vi "CommonVIs_ClassWireSelection.vi"(3 "Offset(-300,0)":T1={"Left"=-231, "Top"=18}, 4 "SaveChangesInClassRightAway(True)":bool=TRUE, 5 "WireStyleSelected":refnum<user-event>, 7 "SelectedWireStyle":refnum<vi>, 8 "error in (no error)":errorcluster, 9 "Messages(Stop or Empty string will stop this VI)":refnum<user-event>, 10 "WireSelectionList":refnum<vi>, 11 "LVClassToActOn":refnum<vi>) -> ()   [LabVIEW 2020]
uses:
  <vilib>/Utility/miscctls.llb/LVPositionTypeDef.ctl
  <resource>/Framework/Providers/Open_GDS/SubVIs/GOOP_WireConfigurationType.ctl
  <resource>/Framework/Providers/Open_GDS/SubVIs/GOOP_WirePattern.ctl
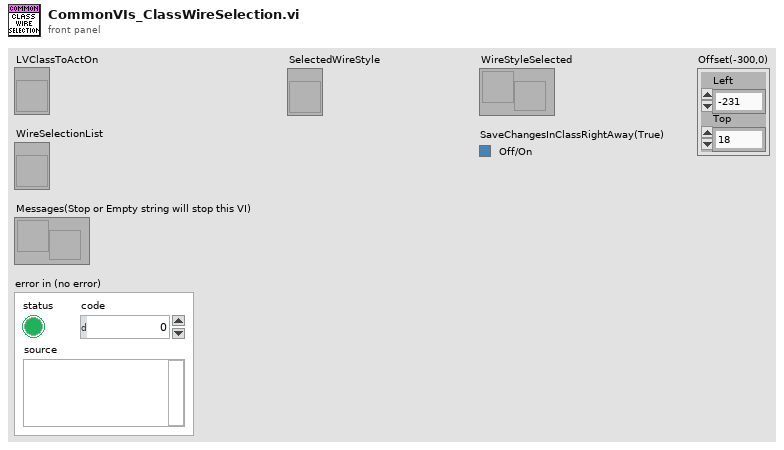
[diagram p1: front panel]
types:
  T1 = typedef "LVPositionTypeDef.ctl" = cluster{"Left":i32, "Top":i32}
  T2 = typedef "GOOP_WireConfigurationType.ctl" = cluster{"Edge thickness":i32, "Edge color":u32, "Center thickness":i32, "Center pattern":T3, "CenterColor1":u32, "CenterColor2":u32, "Tunnels and terminals colors":u32}
  T3 = typedef "GOOP_WirePattern.ctl" = enum16{"Solid", "Large dash", "Small dash"}
  T4 = cluster{"SelectedWireStyle":string, "IconSelection":picture, "CurrentWire":picture, "Icons":string[][], "MarkedIconSelection":picture, "Timeout":i32, "SelectedWireStyle":T2}
  T5 = cluster{"Width":i16, "Style":enum32{"Solid", "Dash", "Dot", "DashDot", "DashDotDot"}}
  T6 = cluster{"left":i16, "top":i16, "right":i16, "bottom":i16}
  T7 = cluster{"IconDimensions":i16, "IconDimensions":i16}
  T8 = cluster{"Foreground Color":u32, "Background Color":u32, "Fill Pattern":cluster{"Row 0":u8, "Row 1":u8, "Row 2":u8, "Row 3":u8, "Row 4":u8, "Row 5":u8, "Row 6":u8, "Row 7":u8}, "Width":i16, "Mode":enum16{"Copy", "Or", "Exclusive Or", "Bit Clear", "Not Copy", "Not Or", "Nor Exclusive Or", "Not Bit Clear"}, "Style":enum32{"Solid", "Dash", "Dot", "Dash Dot", "Dash Dot Dot"}, "Fill Rule":enum32{"Even Odd", "Winding"}, "End Caps":enum32{"Default", "Flat"}}[]
  T9 = typedef "lveventtype.ctl" = enum32{"Null", "Timeout", "Annotation Menu Selection", "Annotation Menu Selection?", "App Instance Close", "App Instance Close?", "Autoscale Range Change", "Bookmark Info Change", "Cell Edit", "Cell Edit?", "Cursor Grab", "Cursor Grab?", "Cursor Menu Selection", "Cursor Menu Selection?", "Cursor Move", "Cursor Release", "Data Change", "Direction Change", "Display State Change", "Drag Ended", "Drag Enter", "Drag Leave", "Drag Over", "Drag Source Update", "Drag Starting", "Drag Starting?", "Drop", "Exec State Change", "Key Down", "Key Down?", "Key Repeat", "Key Repeat?", "Key Up", "Listbox Double Click", "Menu Activation?", "Menu Selection (App)", "Menu Selection? (App)", "Menu Selection (User)", "Mouse Down", "Mouse Down?", "Mouse Enter", "Mouse Leave", "Mouse Move", "Mouse Up", "Mouse Wheel", "NI Security User Change (App)", "Pane Size", "Panel Close", "Panel Close?", "Panel Resize", "Plot Attribute Change", "Scale Range Change", "Shortcut Menu Activation?", "Shortcut Menu Selection (App)", "Shortcut Menu Selection? (App)", "Shortcut Menu Selection (User)", "Tree Double Click", "Tree Drag", "Tree Drag?", "Tree Drop", "Tree Drop?", "Tree Item Close", "Tree Item Close?", "Tree Item Open", "Tree Item Open?", "User Event", "Value Change"}
  T10 = cluster{"IconDimensions":i16, "IconDimensions":i16, "IconDimensions":i16, "IconDimensions":i16}
  T11 = cluster{"IconDimensions":dbl, "IconDimensions":dbl}
  T12 = cluster{"IconDimensions":i32, "IconDimensions":i32}
  T13 = cluster{"IconDimensions":i32, "IconDimensions":i32, "IconDimensions":i32, "IconDimensions":i32}
  T14 = typedef "Scripting_ConnectorPanePatternType.ctl" = u16
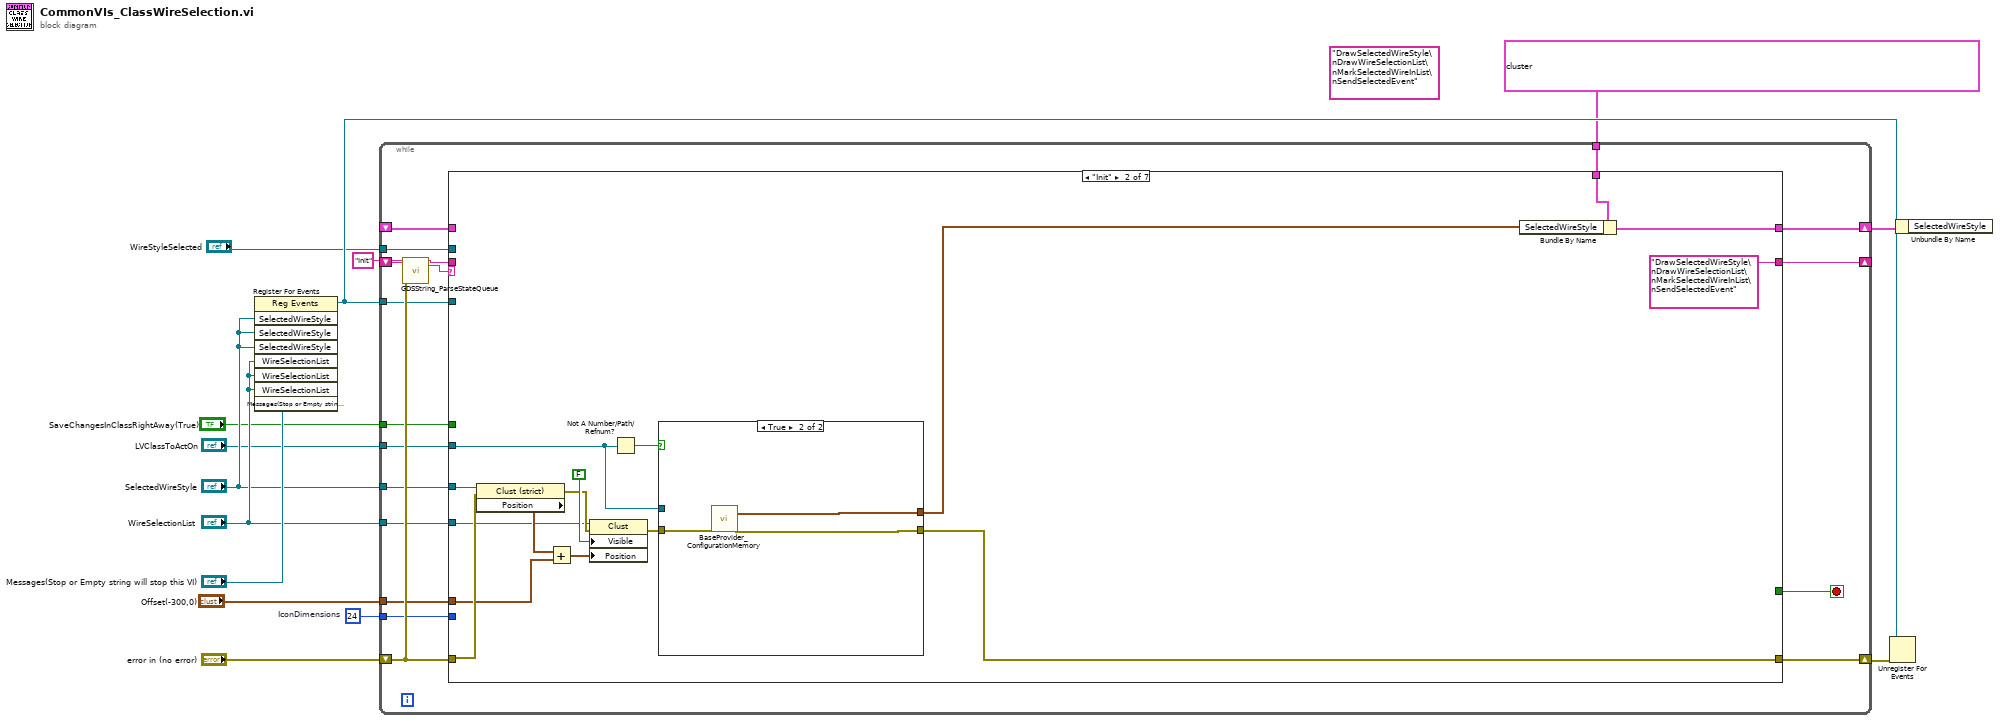
[diagram p0: block diagram]
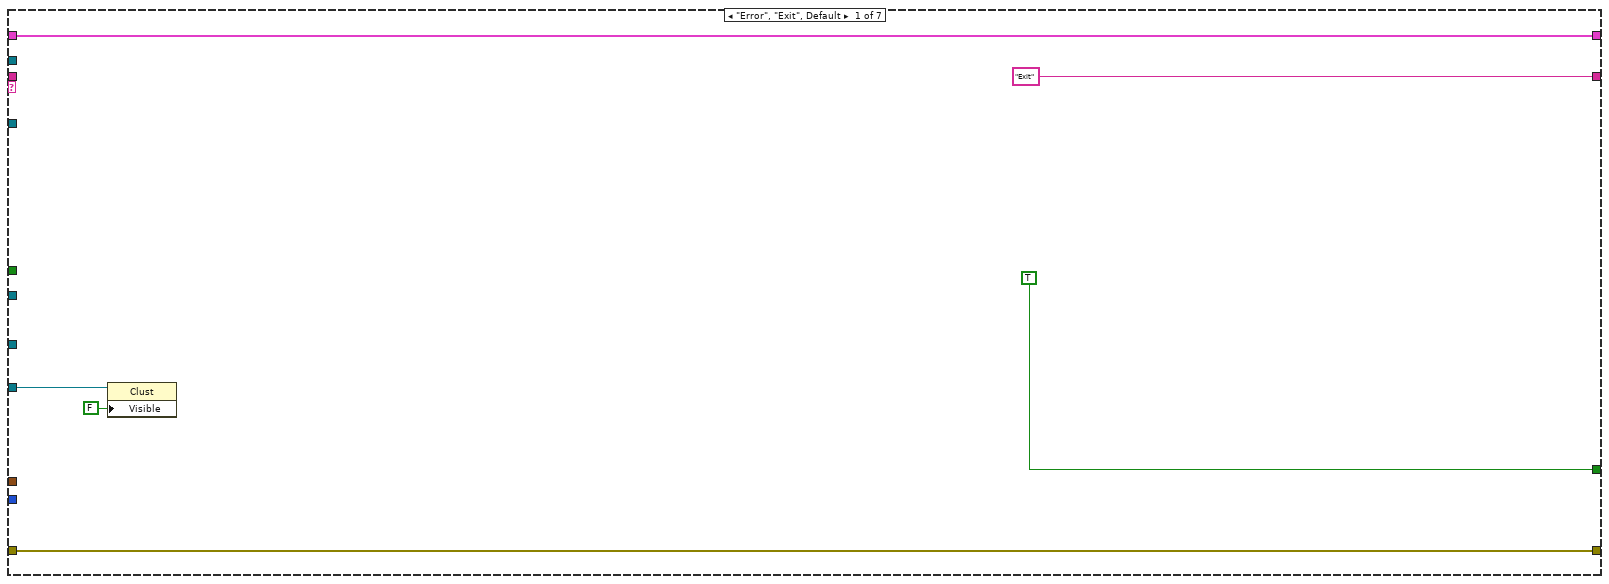
[diagram p2: hidden frame]
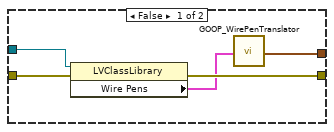
[diagram p3: hidden frame]
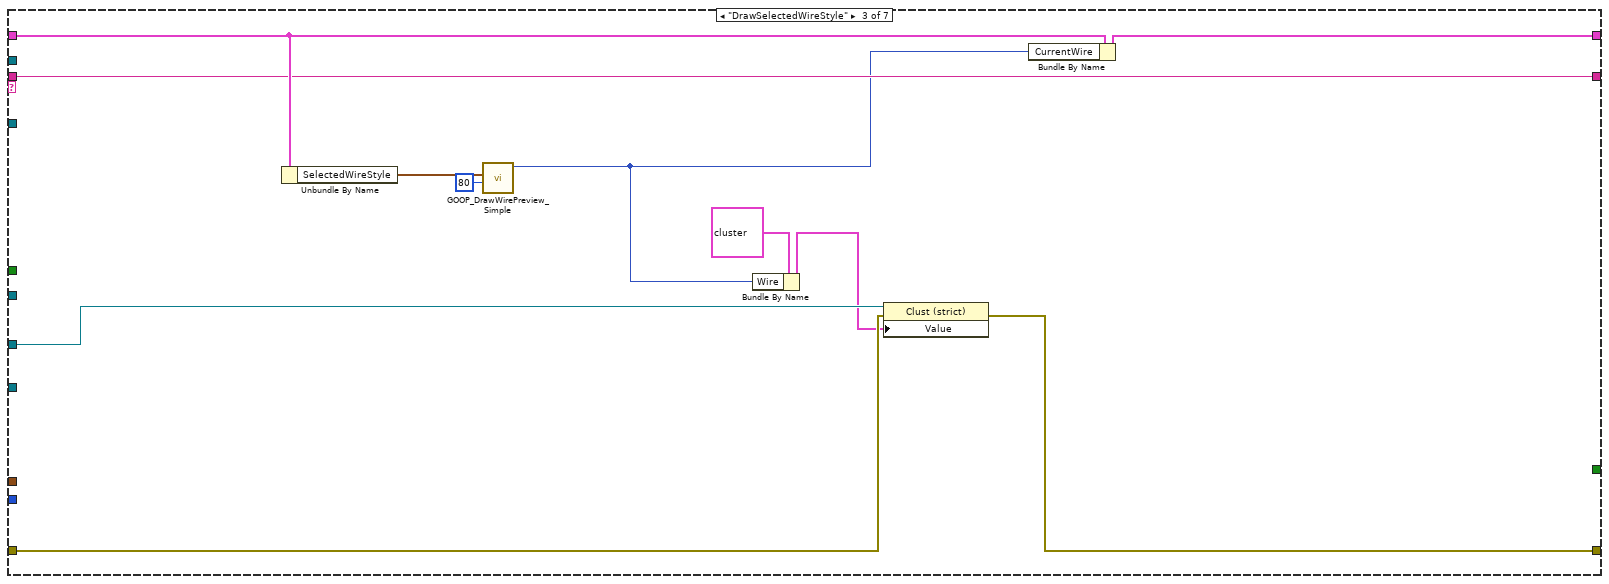
[diagram p4: hidden frame]
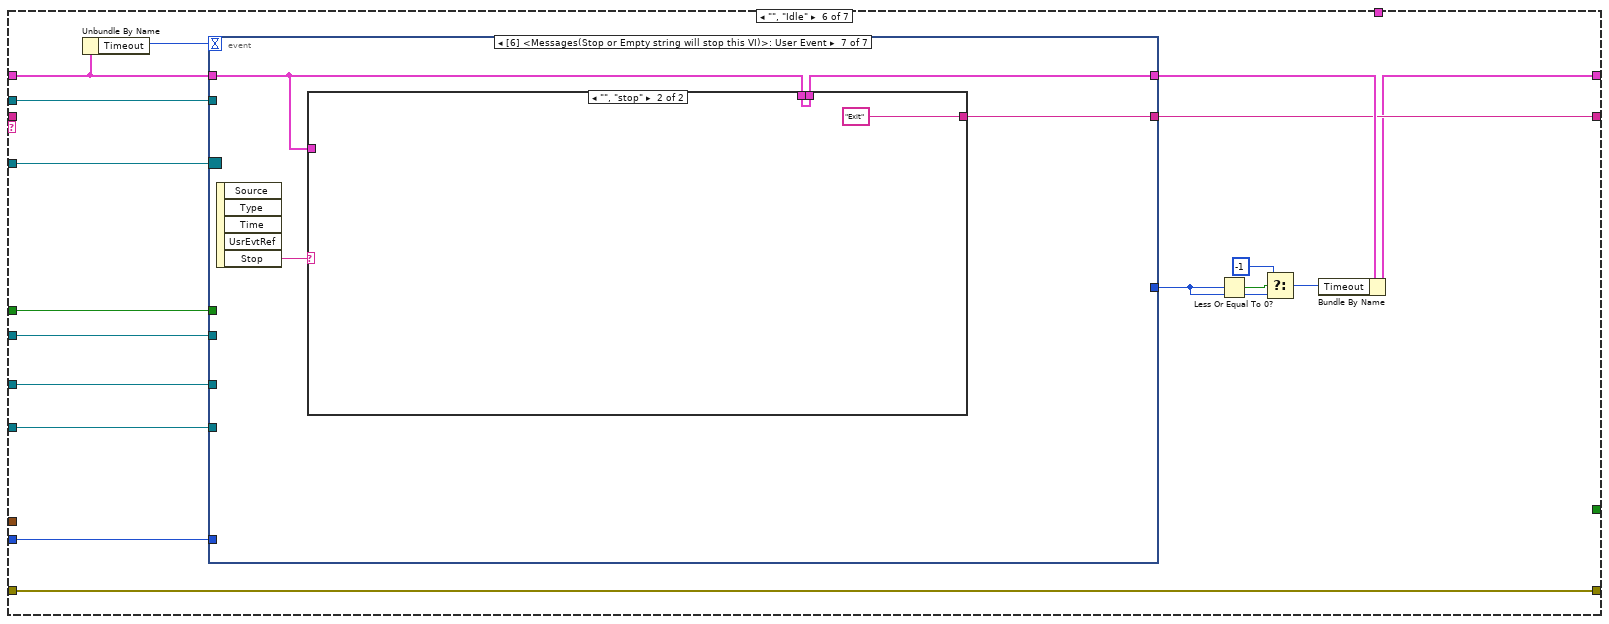
[diagram p7: hidden frame]
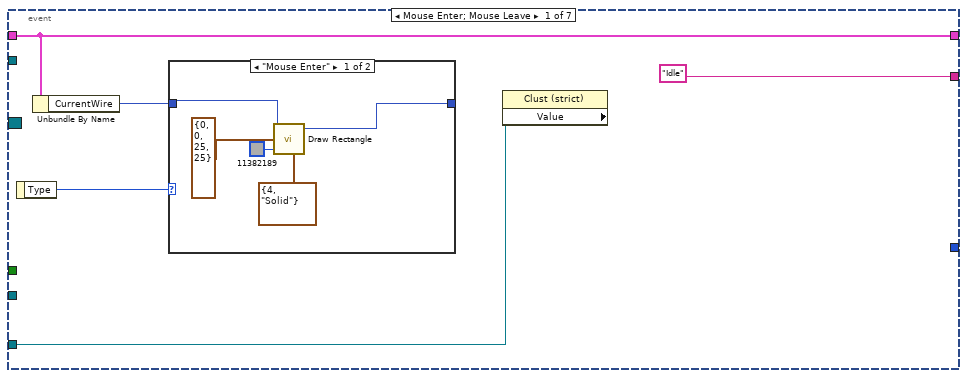
[diagram p8: hidden frame]
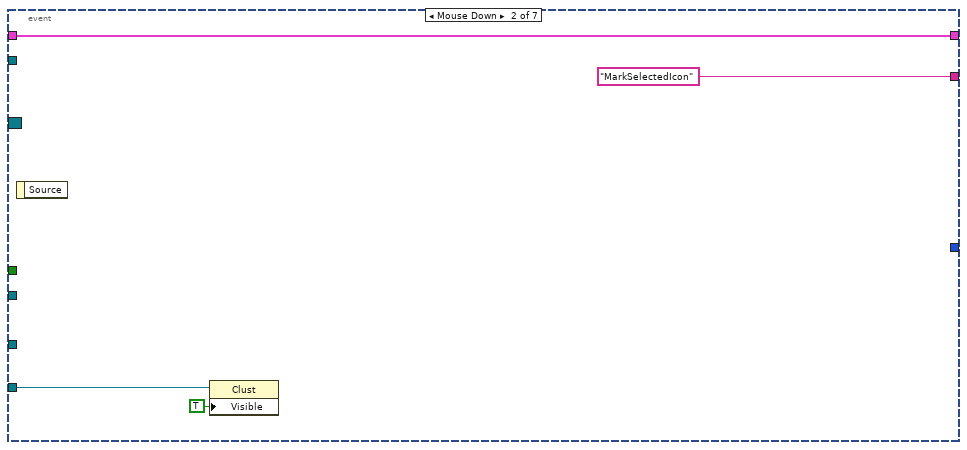
[diagram p10: hidden frame]
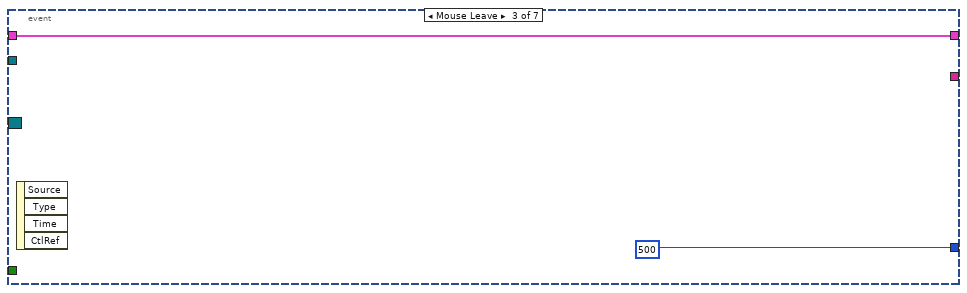
[diagram p11: hidden frame]
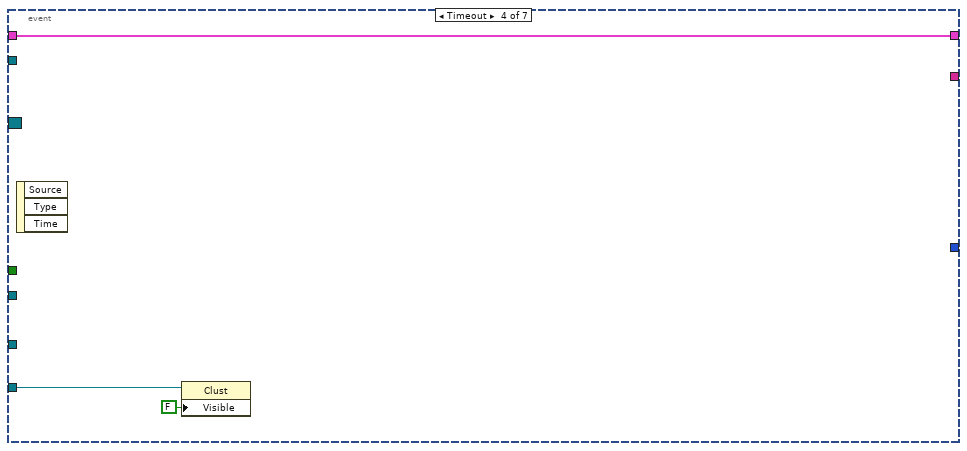
[diagram p12: hidden frame]
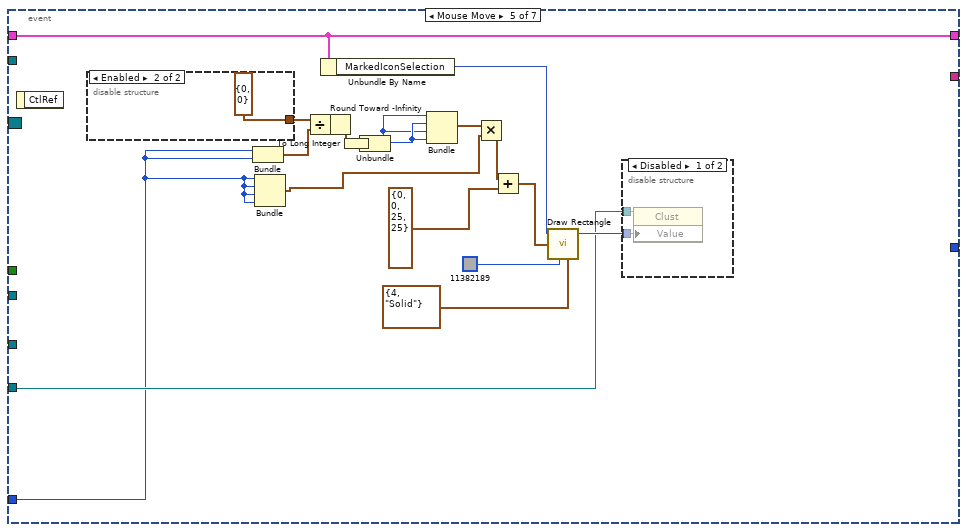
[diagram p13: hidden frame]
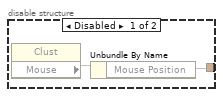
[diagram p15: hidden frame]
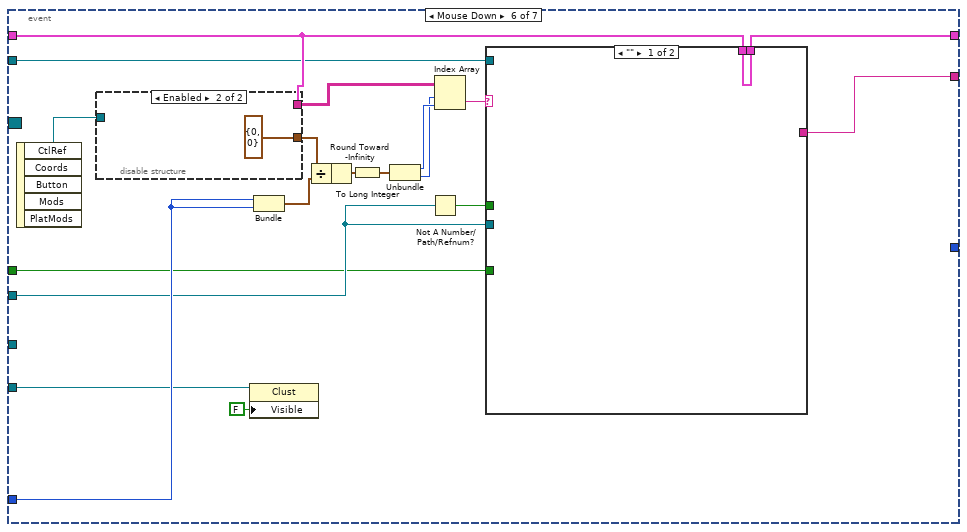
[diagram p16: hidden frame]
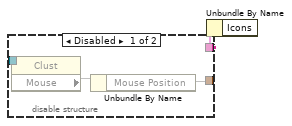
[diagram p17: hidden frame]
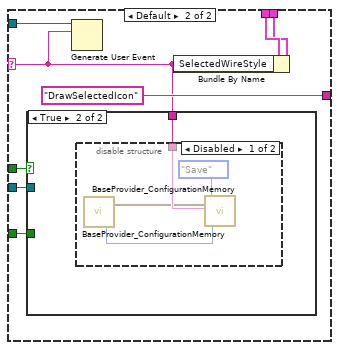
[diagram p18: hidden frame]
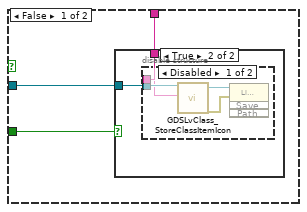
[diagram p19: hidden frame]
diagram:
  (unwired) "DrawSelectedWireStyle\nDrawWireSelectionList\nMarkSelectedWireInList\nSendSelectedEvent"
  w7 = i16 24  # IconDimensions
  n1 = register-events("SelectedWireStyle", "SelectedWireStyle", "SelectedWireStyle", "WireSelectionList", "WireSelectionList", "WireSelectionList", "Messages(Stop or Empty string will stop this VI)") -> (reference out=w11:refnum<event-registration>)  [unwired: 2 in, 1 out]
  n2 = while {
    shift-right: [w28] -> w10
    shift-left: "error in (no error)" -> [w31]
    shift-right: [w27] -> _
    shift-left: "Init" -> [w32]
    tunnel: "WireSelectionList" -> [w30]
    tunnel: "SelectedWireStyle" -> [w29]
    tunnel: w7 -> [w23]
    tunnel: T4 {"SelectedWireStyle"="", "IconSelection"=bytes[0], "CurrentWire"=bytes[0], "Icons"=[], "MarkedIconSelection"=bytes[0], "Timeout"=-1, "SelectedWireStyle"={"Edge thickness"=1, "Edge color"=5667411, "Center thickness"=1, "Center pattern"=enum."Solid", "CenterColor1"=9740924, "CenterColor2"=8694662, "Tunnels and terminals colors"=131187}} -> [w22]
    shift-right: [w21] -> w13
    shift-left: _ -> [w20]
    tunnel: w11 -> [w19]
    tunnel: "LVClassToActOn" -> [w18]
    tunnel: "WireStyleSelected" -> [w17]
    tunnel: "SaveChangesInClassRightAway(True)" -> [w16]
    tunnel: "Offset(-300,0)" -> [w15]
    stop <- w26 stop-if-true
    n3 = call <resource>:"GDSString_ParseStateQueue.vi"("State Queue"=w32, "Error In (no error)"=w31) -> ("Remaining States"=w25:string, "Current State"=w24:string)  [unwired: 9 in, 3 out]
    n4 = case shown="\"Init\"" w24 {
      tunnel: w31 -> [w38 w52 w67 w76 w78 w96 w216]
      tunnel: w30 -> [w34 w46 _ _ _ w92 _]
      tunnel: w29 -> [_ w47 w69 _ _ w83 _]
      tunnel: [w38 w45 w72 w76 w78 w96 w216] -> w28
      tunnel: ["Exit" "DrawSelectedWireStyle\nDrawWireSelectionList\nMarkSelectedWireInList\nSendSelectedEvent" w70 w75 w79 w93 w215] -> w27
      tunnel: [TRUE _ _ _ _ _ _] -> w26
      tunnel: w25 -> [_ _ w70 w75 w79 _ w215]
      tunnel: w23 -> [_ _ _ _ _ w91 _]
      tunnel: w22 -> [_ w49 _ _ _ _ _]
      tunnel: [w35 w48 w71 w74 w77 w90 w213] -> w21
      tunnel: w20 -> [w35 _ w73 w74 w77 w85 w213]
      tunnel: w19 -> [_ _ _ _ _ w95 _]
      tunnel: w18 -> [_ w42 _ _ _ w82 _]
      tunnel: w17 -> [_ _ _ _ _ w81 w214]
      tunnel: w16 -> [_ _ _ _ _ w80 _]
      tunnel: w15 -> [_ w39 _ _ _ _ _]
      frame "Error", "Exit", Default {
        n5 = property class="Clust"(reference=w34, "Visible"=FALSE) -> ()  [unwired: 1 in, 2 out]
      }
      frame "Init" {
        n6 = property class="Clust (strict)"(reference=w47, error in=w52) -> (error out=w51:errorcluster, "Position"=w54:T1)  [unwired: 1 out]
        n7 = Add(x=w54, y=w39) -> (x+y=w40:T1)
        n8 = property class="Clust"(reference=w46, error in=w51, "Visible"=FALSE, "Position"=w40) -> (error out=w50:errorcluster)  [unwired: 1 out]
        n9 = Not A Number/Path/Refnum?(number/path/refnum=w42) -> (NaN/Path/Refnum?=w43:bool)
        n10 = case shown="True" w43 {
          tunnel: w50 -> [w58 w62]
          tunnel: [w57 w61] -> w45
          tunnel: [w56 w60] -> w44
          tunnel: w42 -> [w59 _]
          frame False {
            n11 = property class="LVClassLibrary"(reference=w59, error in=w58) -> (error out=w57:errorcluster, "Wire Pens"=w55:T8)  [unwired: 1 out]
            n12 = call <resource>:"GOOP_WirePenTranslator.vi"("WirePensIn"=w55) -> ("WireConfigurationOut"=w56:T2)  [unwired: 17 in, 1 out]
          }
          frame True {
            n13 = call <resource>:"BaseProvider_ConfigurationMemory.vi"("error in (no error)"=w62) -> ("WireConfigurationOut"=w60:T2, "error out"=w61:errorcluster)  [unwired: 12 in, 5 out]
          }
        }
        n14 = Bundle By Name(cluster=w49, "SelectedWireStyle"=w44) -> (w48:T4)
      }
      frame "DrawSelectedWireStyle" {
        n15 = Unbundle By Name(w73) -> ("SelectedWireStyle"=w68:T2)
        n16 = call <resource>:"GOOP_DrawWirePreview_Simple.vi"("WireLength(100px)"=i16 80, "WireConfiguration"=w68) -> ("WirePictureOut"=w64:picture)  [unwired: 5 in, 4 out]
        n17 = Bundle By Name(cluster=cluster{"Name":string, "Wire":picture} {"Name"="Default", "Wire"=bytes[0]} ("Value"), "Wire"=w64) -> (w65:cluster{"Name":string, "Wire":picture})
        n18 = property class="Clust (strict)"(reference=w69, error in=w67, "Value"=w65) -> (error out=w72:errorcluster)  [unwired: 1 out]
        n19 = Bundle By Name(cluster=w73, "CurrentWire"=w64) -> (w71:T4)
      }
      frame "DrawWireSelectionList" {
      }
      frame "MarkSelectedWireInList" {
      }
      frame "", "Idle" {
        n20 = Unbundle By Name(w85) -> ("Timeout"=w84:i32)
        n21 = event shown="[6] <Messages(Stop or Empty string will stop this VI)>: User Event" {
          selector: w95 -> [_ _ _ _ _ _ _]
          dyn-events: _ -> [_ _ _ _ _ _ _]
          timeout: w84 -> [_ _ _ _ _ _ _]
          tunnel: w85 -> [w100 w109 w113 w116 w122 w153 w190]
          tunnel: [w100 w109 w113 w116 w122 w151 w191] -> w94
          tunnel: ["Idle" "MarkSelectedIcon" _ _ _ w149 w192] -> w93
          tunnel: w92 -> [_ w111 _ w114 w119 w147 _]
          tunnel: w91 -> [_ _ _ _ w118 w154 _]
          tunnel: [_ _ 500 ("500") _ _ _ _] -> w87
          tunnel: w83 -> [w97 _ _ _ _ _ _]
          tunnel: w82 -> [_ _ _ _ _ w143 _]
          tunnel: w81 -> [_ _ _ _ _ w142 _]
          tunnel: w80 -> [_ _ _ _ _ w141 _]
          event Mouse Enter; Mouse Leave {
            n22 = event-data() -> ("Type"=w101:T9)  [unwired: 1 in]
            n23 = Unbundle By Name(w100) -> ("CurrentWire"=w99:picture)
            n24 = case shown="\"Mouse Enter\"" w101 {
              tunnel: [w104 w107] -> _
              tunnel: w99 -> [w103 w107]
              frame "Mouse Enter" {
                n25 = call <vilib>:"Draw Rectangle.vi"("picture"=w103, "rect"=T6 {"left"=0, "top"=0, "right"=25, "bottom"=25}, "color(black)"=u32 11382189, "pen"=T5 {"Width"=4, "Style"=enum."Solid"}) -> ("new picture"=w104:picture)  [unwired: 5 in]
              }
              frame "Mouse Leave", Default {
              }
            }
            n26 = property class="Clust (strict)" props=["Value"](reference=w97) -> ()  [unwired: 1 in, 3 out]
          }
          event Mouse Down {
            n27 = event-data() -> ()  [unwired: 1 in, 1 out]
            n28 = property class="Clust"(reference=w111, "Visible"=TRUE) -> ()  [unwired: 1 in, 2 out]
          }
          event Mouse Leave {
            n29 = event-data() -> ()  [unwired: 1 in, 4 out]
          }
          event Timeout {
            n30 = event-data() -> ()  [unwired: 1 in, 3 out]
            n31 = property class="Clust"(reference=w114, "Visible"=FALSE) -> ()  [unwired: 1 in, 2 out]
          }
          event Mouse Move {
            n32 = event-data() -> ()  [unwired: 1 in, 1 out]
            n33 = disable-structure shown="Enabled" {
              disable-tunnel: [w139 T7 {"IconDimensions"=0, "IconDimensions"=0} ("x")] -> w124
              frame Disabled {
                n34 = property on="Property Node" class="Clust"() -> ("Mouse"=w138)  [unwired: 2 in, 2 out]
                n35 = Unbundle By Name(w138) -> ("Mouse Position"=w139)
              }
              frame Enabled {
              }
            }
            n36 = Bundle("IconDimensions"=w118, "IconDimensions"=w118) -> (w123:T7)  [unwired: 1 in]
            n37 = Bundle("IconDimensions"=w118, "IconDimensions"=w118, "IconDimensions"=w118, "IconDimensions"=w118) -> (w117:T10)  [unwired: 1 in]
            n38 = Divide(x=w124, y=w123) -> (x/y=w125:T11)
            n39 = Unbundle By Name(w122) -> ("MarkedIconSelection"=w121:picture)
            n40 = Round Toward -Infinity(1:w125) -> (0:w126:T11)
            n41 = To Long Integer(number=w126) -> (32bit integer=w131:T12)
            n42 = Unbundle(w131) -> ("IconDimensions"=w129:i32, "IconDimensions"=w130:i32)
            n43 = Bundle("IconDimensions"=w129, "IconDimensions"=w130, "IconDimensions"=w129, "IconDimensions"=w130) -> (w132:T13)  [unwired: 1 in]
            n44 = Multiply(x=w132, y=w117) -> (x*y=w134:T13)
            n45 = Add(x=w134, y=T6 {"left"=0, "top"=0, "right"=25, "bottom"=25} ("rect")) -> (x+y=w135:cluster{i32, i32, i32, i32})
            n46 = call <vilib>:"Draw Rectangle.vi"("picture"=w121, "rect"=w135, "color(black)"=u32 11382189, "pen"=T5 {"Width"=4, "Style"=enum."Solid"}) -> ("new picture"=w120:picture)  [unwired: 5 in]
            n47 = disable-structure shown="Disabled" {
              disable-tunnel: w120 -> [w137 _]
              disable-tunnel: w119 -> [w136 _]
              frame Disabled {
                n48 = property class="Clust"(reference=w136, "Value"=w137) -> ()  [unwired: 1 in, 2 out]
              }
              frame Enabled {
              }
            }
          }
          event Mouse Down {
            n49 = event-data() -> ("CtlRef"=w155:refnum<vi>)  [unwired: 1 in, 4 out]
            n50 = disable-structure shown="Enabled" {
              disable-tunnel: [w165 T7 {"IconDimensions"=0, "IconDimensions"=0} ("x")] -> w157
              disable-tunnel: w155 -> [w163 _]
              disable-tunnel: w153 -> [w162 _]
              disable-tunnel: [w161 _] -> w152
              frame Disabled {
                n51 = property on="Property Node" class="Clust"(reference=w163) -> ("Mouse"=w164)  [unwired: 1 in, 2 out]
                n52 = Unbundle By Name(w164) -> ("Mouse Position"=w165)
                n53 = Unbundle By Name(w162) -> ("Icons"=w161:string[][])
              }
              frame Enabled {
              }
            }
            n54 = property class="Clust"(reference=w147, "Visible"=FALSE) -> ()  [unwired: 1 in, 2 out]
            n55 = Bundle("IconDimensions"=w154, "IconDimensions"=w154) -> (w156:T7)  [unwired: 1 in]
            n56 = Divide(x=w157, y=w156) -> (x/y=w158:T11)
            n57 = Round Toward -Infinity(1:w158) -> (0:w159:T11)
            n58 = To Long Integer(number=w159) -> (32bit integer=w160:T12)
            n59 = Unbundle(w160) -> ("IconDimensions"=w146:i32, "IconDimensions"=w145:i32)
            n60 = Not A Number/Path/Refnum?(number/path/refnum=w143) -> (NaN/Path/Refnum?=w144:bool)
            n61 = Index Array(array=w152, index (row)=w145, index (col)=w146) -> (element=w150:string)
            n62 = case shown="\"\"" w150 {
              selector: w150 -> [_ w170]
              tunnel: w153 -> [w167 w175]
              tunnel: [w167 w174] -> w151
              tunnel: [_ "DrawSelectedIcon"] -> w149
              tunnel: w144 -> [_ w172]
              tunnel: w143 -> [_ w171]
              tunnel: w142 -> [_ w169]
              tunnel: w141 -> [_ w168]
              frame "" {
              }
              frame Default {
                n63 = case shown="True" w172 {
                  tunnel: w170 -> [w177 w185]
                  tunnel: w171 -> [w178 _]
                  tunnel: w168 -> [w176 _]
                  frame False {
                    n64 = case shown="True" w176 {
                      tunnel: w178 -> [_ w180]
                      tunnel: w177 -> [_ w179]
                      frame False {
                      }
                      frame True {
                        n65 = disable-structure shown="Disabled" {
                          disable-tunnel: w180 -> [w184 _]
                          disable-tunnel: w179 -> [w183 _]
                          frame Disabled {
                            n66 = call <resource>:"GDSLvClass_StoreClassItemIcon.vi"("Library Refnum"=w184, "ClassItemIconName"=w183) -> ("Library Refnum"=w182:refnum<vi>, "error out"=w181:errorcluster)  [unwired: 16 in]
                            n67 = invoke class="Library" method="Save"(reference=w182, error in=w181) -> ()  [unwired: 2 in, 4 out]
                          }
                          frame Enabled {
                          }
                        }
                      }
                    }
                  }
                  frame True {
                    n68 = disable-structure shown="Disabled" {
                      disable-tunnel: w185 -> [w189 _]
                      frame Disabled {
                        n69 = call <resource>:"BaseProvider_ConfigurationMemory.vi"() -> ("PatternOut"=w188:T14, "WireConfigurationOut"=w187:T2)  [unwired: 13 in, 5 out]
                        n70 = call <resource>:"BaseProvider_ConfigurationMemory.vi"("WireConfiguration"=w187, "Icon"=w189, "Action"=enum16{"Read", "Load", "Save", "Set"}."Save", "PatternIn"=w188) -> ()  [unwired: 9 in, 7 out]
                      }
                      frame Enabled {
                      }
                    }
                  }
                }
                n71 = Generate User Event(user event=w169, event data cluster=w170) -> ()  [unwired: 2 in, 2 out]
                n72 = Bundle By Name(cluster=w175, "SelectedWireStyle"=w170) -> (w174:T4)
              }
            }
          }
          event User Event {
            n73 = event-data() -> ("Stop"=w193:string)  [unwired: 1 in, 4 out]
            n74 = case shown="\"\", \"stop\"" w193 {
              selector: w193 -> [w197 _]
              tunnel: ["DrawSelectedIcon\nMarkSelectedIcon" "Exit"] -> w192
              tunnel: w190 -> [w204 w210]
              tunnel: [w203 w210] -> w191
              tunnel: w190 -> [w202 _]
              frame Default {
                n75 = Unbundle By Name(w202) -> ("Icons"=w201:string[][], "SelectedWireStyle"=w196:string)
                n76 = To Lower Case(string=w197) -> (all lower case string=w199:string)
                n77 = To Lower Case(string=w201) -> (all lower case string=w200:string[][])
                n78 = for {
                  tunnel: w200 -> [w209] mode=indexing
                  tunnel: w199 -> [w208]
                  tunnel: [w207] -> _
                  tunnel: [w205] -> w198
                  i -> [w207]
                  stop <- w205 stop-if-true
                  n79 = Search 1D Array(1D array=w209, element=w208) -> (index of element=w206:i32)  [unwired: 1 in]
                  n80 = Greater Or Equal To 0?(x=w206) -> (x >= 0?=w205:bool)
                }
                n81 = Select(t=w197, s=w198, f=w196) -> (s? t:f=w195:string)
                n82 = Bundle By Name(cluster=w204, "SelectedWireStyle"=w195) -> (w203:T4)
              }
              frame "", "stop" {
              }
            }
          }
        }
        n83 = Less Or Equal To 0?(x=w87) -> (x <= 0?=w89:bool)
        n84 = Select(t=-1, s=w89, f=w87) -> (s? t:f=w88:i32)
        n85 = Bundle By Name(cluster=w94, "Timeout"=w88) -> (w90:T4)
      }
      frame "SendSelectedEvent" {
        n86 = Unbundle By Name(w213) -> ("SelectedWireStyle"=w212:string)
        n87 = Generate User Event(user event=w214, event data cluster=w212) -> ()  [unwired: 2 in, 2 out]
      }
    }
  }
  n88 = Unregister For Events(event registration refnum=w11, error in=w10) -> ()  [unwired: 1 out]
  n89 = Unbundle By Name(w13) -> ()  [unwired: 1 out]
